vi "Filter NICs.vi"(8 "Error In":errorcluster, 10 "NIC Name":string="lo", 11 "NIC Configs":T1[](array[typedef])) -> (0 "Error Out":errorcluster, 3 "NIC Configs":T1[](array[typedef]))   [LabVIEW 2020, in "LMH-LINX.lvlib"]
uses:
  LMH-LINX.lvlib
  NIC Info.ctl
  NIC Mode.ctl
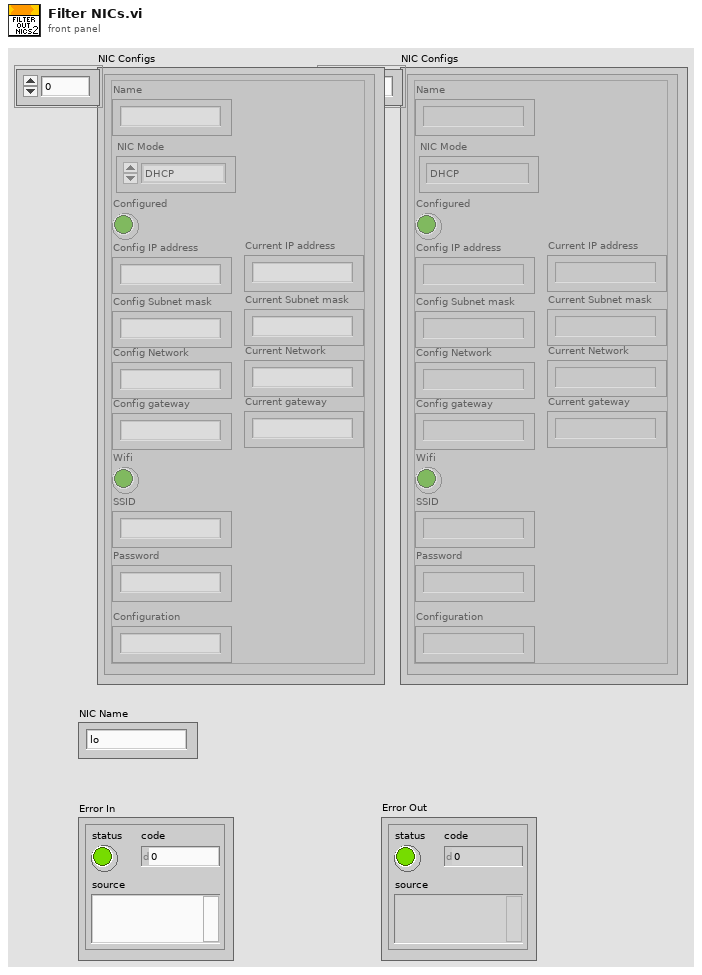
[diagram p1: front panel]
types:
  T1 = typedef "LMH-LINX.lvlib/NIC Info.ctl" = cluster{"Name":string, "NIC Mode":T2, "Configured":bool, "Config IP address":string, "Config Subnet mask":string, "Config Network":string, "Config gateway":string, "Wifi":bool, "SSID":string, "Password":string, "Configuration":string, "Current IP address":string, "Current Subnet mask":string, "Current gateway":string, "Current Network":string}
  T2 = typedef "LMH-LINX.lvlib/NIC Mode.ctl" = enum16{"DHCP", "Static", "Loopback"}
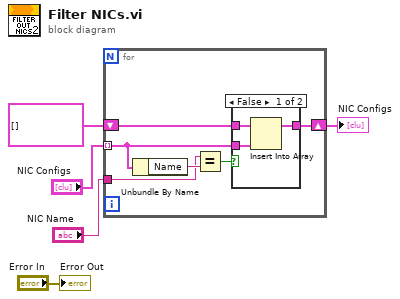
[diagram p0: block diagram]
diagram:
  n1 = for {
    tunnel: "NIC Configs" -> [w7] mode=indexing
    shift-right: [w8] -> w5
    shift-left: T1[] [] ("NIC Configs") -> [w9]
    tunnel: "NIC Name" -> [w6]
    n2 = Unbundle By Name(w7) -> ("Name"=w11:string)
    n3 = Equal?(x=w6, y=w11) -> (x = y?=w10:bool)
    n4 = case shown="False" w10 {
      tunnel: w9 -> [w14 w15]
      tunnel: [w13 w15] -> w8
      tunnel: w7 -> [w12 _]
      frame False {
        n5 = Insert Into Array(array=w14, new element=w12) -> (w13:T1[])  [unwired: 1 in]
      }
      frame True {
      }
    }
  }
  "NIC Configs" <- w5
  "Error Out" <- "Error In"
